vi "FreqInit2FreqFinal.vi"(3 "entrée d'erreur":errorcluster, 4 "NomProjet":string, 5 "CheminFichier":path) -> (0 "sortie d'erreur":errorcluster, 2 "chemin du fichier en sortie":path)   [LabVIEW 2015]
uses:
  <vilib>/Analysis/NI_AALBase.lvlib
  <vilib>/Analysis/baseanly.llb/Mean (DBL).vi
panel:
  out "taille(s) 3":i32
  out "taille(s) 2":i32
  out "taille(s)":i32
  out "DonnesOrigine":waveform(dbl)[](graph)
  out "DonnesFinales":waveform(dbl)[](graph)
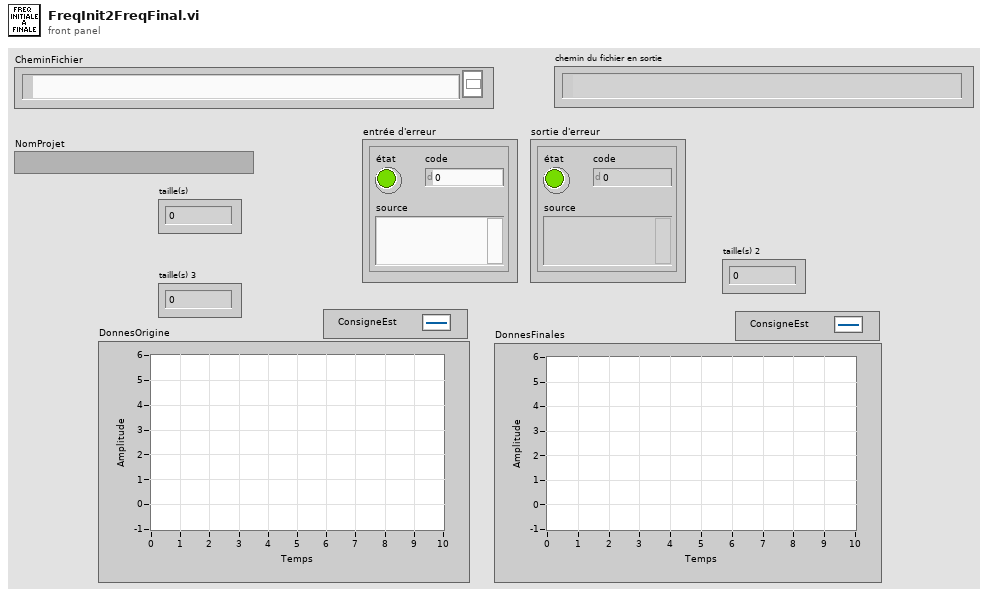
[diagram p1: front panel]
types:
  T1 = enum16{"open", "open or create", "create or replace", "create", "open (read-only)"}
  T2 = typedef "ConfigMesuresPCServeur.ctl" = cluster{"ChannelsNb":u32, "SamplingRate (Hz)":u32, "AcquisitionTime (s)":u32, "External Trigger":bool, "Final Sampl. Rate (Hz)":u32, "Channel names":string[], "Channel units":string[], "Gains":dbl[], "Offset":dbl[], "TareAuto":bool[], "1ere voie balance":u32, "Quelle balance?":T3, "Batch Capture":bool, "Dossier BackUP":path}
  T3 = typedef "QuelleBalance.ctl" = enum16{"Pas de balance", "Sixaxes6comp150DaN", "AMTI-UDW3", "PiezoKistler"}
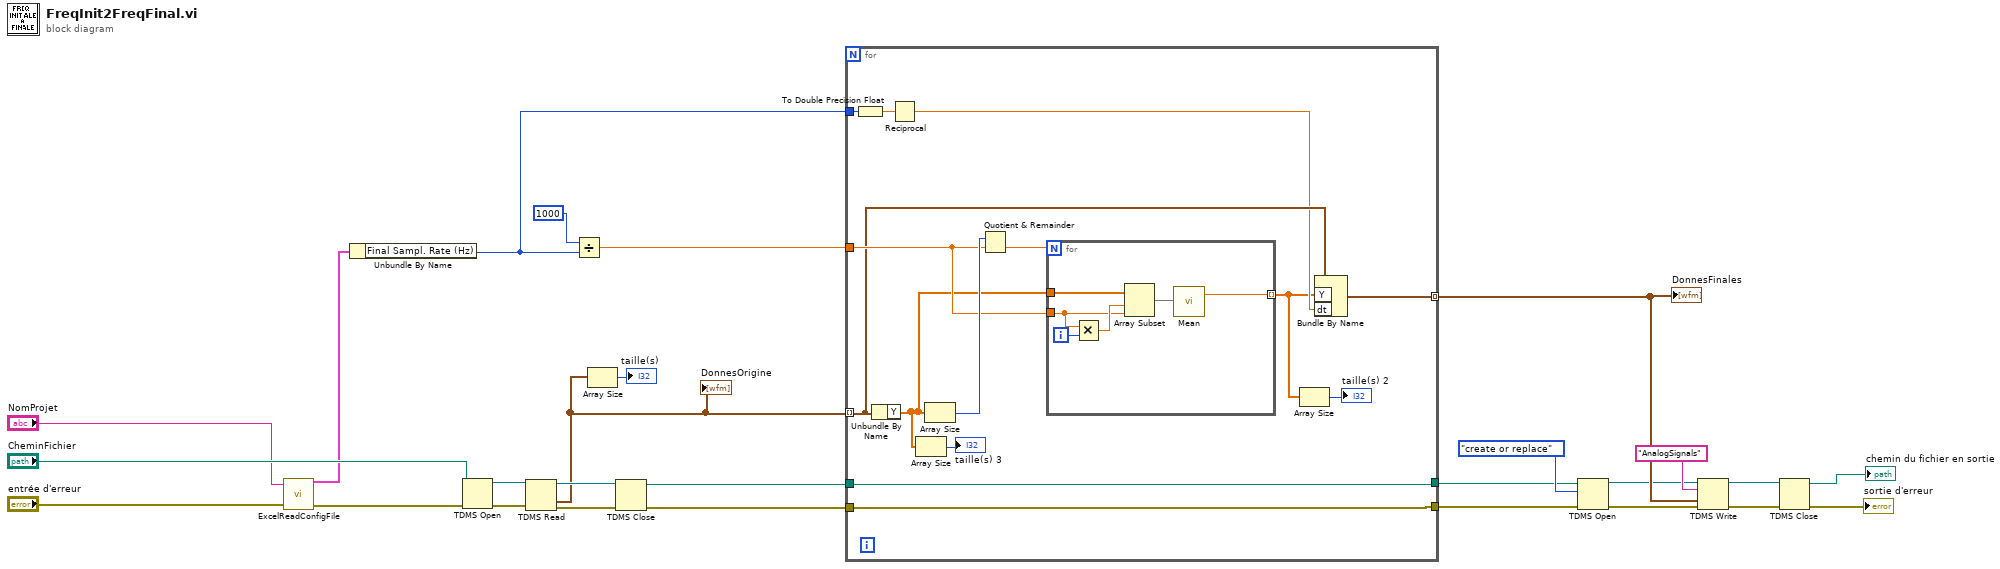
[diagram p0: block diagram]
diagram:
  n1 = call "ExcelReadConfigFile.vi"("error in (no error)"="entrée d'erreur", "NomProjet"="NomProjet") -> ("error out"=w11:errorcluster, "ConfigMesuresPCServeur"=w4:T2)  [unwired: 2 in]
  n2 = Unbundle By Name(w4) -> ("Final Sampl. Rate (Hz)"=w2:u32)
  n3 = TDMS Open(8:w11, 11:"CheminFichier") -> (0:w15:errorcluster, 3:w14:refnum<k34>)  [unwired: 5 in]
  n4 = TDMS Read(0:w14, 11:w15) -> (4:w21:refnum<k34>, 10:w17:waveform(dbl)[], 15:w20:errorcluster)  [unwired: 6 in, 3 out]
  "DonnesOrigine" <- w17
  n5 = Divide(x=u32 1000, y=w2) -> (x/y=w3:dbl)
  n6 = Array Size(array=w17) -> (size(s)=→"taille(s)":i32)
  n7 = TDMS Close(8:w20, 11:w21) -> (0:w18:errorcluster, 3:w10:path)
  n8 = for {
    tunnel: w17 -> [w38] mode=indexing
    tunnel: w18 -> [w35]
    tunnel: [w35] -> w5
    tunnel: [w37] -> w23 mode=indexing
    tunnel: w10 -> [w36]
    tunnel: [w36] -> w6
    tunnel: w3 -> [w39]
    tunnel: w2 -> [w34]
    n9 = To Double Precision Float(number=w34) -> (double precision float=w28:dbl)
    n10 = Unbundle By Name(w38) -> ("Y"=w30:dbl[])
    n11 = Reciprocal(x=w28) -> (1/x=w33:dbl)
    n12 = Array Size(array=w30) -> (size(s)=→"taille(s) 3":i32)
    n13 = Array Size(array=w30) -> (size(s)=w41:i32)
    n14 = Quotient & Remainder(x=w41, y=w39) -> (floor(x/y)=w40:dbl)  [unwired: 1 out]
    n15 = for {
      N: w40 -> [_]
      tunnel: w39 -> [w45]
      tunnel: w30 -> [w44]
      tunnel: [w42] -> w32 mode=indexing
      i -> [w47]
      n16 = Multiply(x=w45, y=w47) -> (x*y=w46:dbl)
      n17 = Array Subset(array=w44, index=w46, length=w45) -> (w43:dbl[])
      n18 = call-poly <vilib>:"Mean.vi"("X"=w43) -> ("mean"=w42:dbl)  [unwired: 1 out]
    }
    n19 = Array Size(array=w32) -> (size(s)=→"taille(s) 2":i32)
    n20 = Bundle By Name(cluster=w38, "Y"=w32, "dt"=w33) -> (w37:waveform(dbl))
  }
  "DonnesFinales" <- w23
  n21 = TDMS Open(8:w5, 10:T1."create or replace" ("opération (0 : open)"), 11:w6) -> (0:w12:errorcluster, 3:w13:refnum<k34>)  [unwired: 4 in]
  n22 = TDMS Write(0:w13, 5:"AnalogSignals" ("nom du groupe en entrée (Sans titre)"), 9:w23, 11:w12) -> (4:w27:refnum<k34>, 15:w26:errorcluster)  [unwired: 2 in, 2 out]
  n23 = TDMS Close(8:w26, 11:w27) -> (0:→"sortie d'erreur":errorcluster, 3:→"chemin du fichier en sortie":path)
